vi "Read instanceVIRef.vi"(8 "error in (no error)":errorcluster, 11 "PolymorphicInstance in":refnum<class "PolymorphicInstance.lvclass">) -> (0 "error out":errorcluster, 2 "instanceVIRef":refnum<vi>, 3 "PolymorphicInstance out":refnum<class "PolymorphicInstance.lvclass">)   [LabVIEW 2012, in "PolymorphicInstance.lvclass"]
uses:
  PolymorphicInstance.lvclass
  PolymorphicInstance.lvclass/PolymorphicInstance.ctl
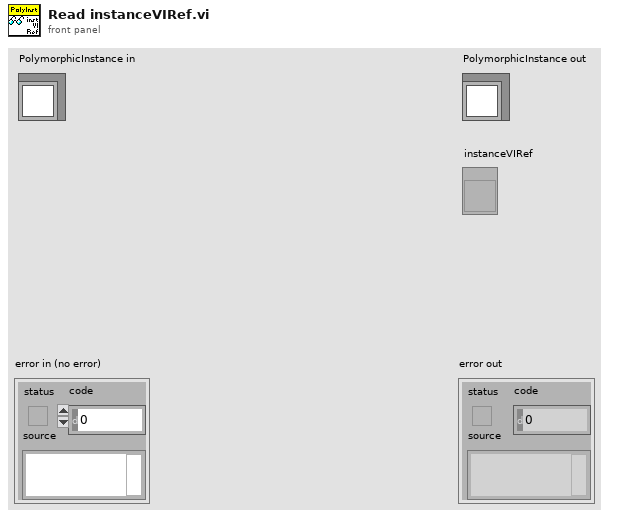
[diagram p1: front panel]
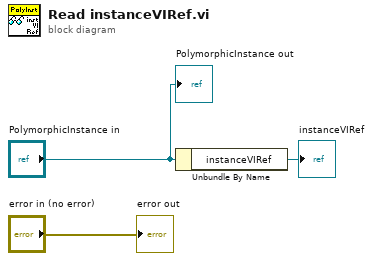
[diagram p0: block diagram]
diagram:
  n1 = Unbundle By Name("PolymorphicInstance in") -> ("instanceVIRef"=→"instanceVIRef":refnum<vi>)
  "error out" <- "error in (no error)"
  "PolymorphicInstance out" <- "PolymorphicInstance in"
